vi "Do Move.vi"(7 "Team in":refnum<class "Team.lvclass">, 10 "Position":T1, 11 "Square in":refnum<class "Square.lvclass">) -> (3 "Square out":refnum<class "Square.lvclass">, 5 "Team out":refnum<class "Team.lvclass">)   [LabVIEW 2020, in "SquareBattle.lvlib" / "Square.lvclass"]
uses:
  Square.lvclass
  Team/Team.lvclass
  Position.ctl
  Square.lvclass/Square.ctl
  SquareBattle.lvlib
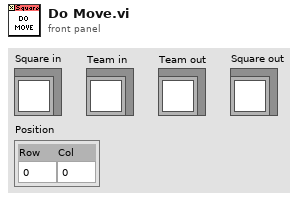
[diagram p1: front panel]
types:
  T1 = typedef "SquareBattle.lvlib/Position.ctl" = cluster{"Row":i32, "Col":i32}
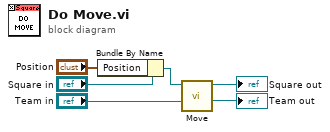
[diagram p0: block diagram]
diagram:
  n1 = Bundle By Name(cluster="Square in", "Position"="Position") -> (w4:refnum<class "Square.lvclass">)
  n2 = call-dynamic "Move.vi"("Team In"="Team in", "Square in"=w4) -> ("Team"=→"Team out":refnum<class "Team.lvclass">, "Square out"=→"Square out":refnum<class "Square.lvclass">)  [unwired: 8 in]
